vi "Parse Core.vi"(0 "SA Path in":refnum<class "SA 18GHz Path.lvclass">, 5 "Config Row":string[](array[string]), 11 "error in":errorcluster) -> (4 "SA Path out":refnum<class "SA 18GHz Path.lvclass">, 15 "error out":errorcluster)   [LabVIEW 2023, in "RFFixtureCharact.RFPM.lvlib" / "SA 18GHz Path.lvclass"]
uses:
  SA 18GHz Path.lvclass
  C:/srd-semi-rfcal-software/AuxTools/STSRFFixtureCharactUtility/Source/Code Modules/Common/Base Classes/Path/Path.lvclass
  Charact Result Accessor/Scalar/Scalar Charact Result Accessor.lvclass
  C:/srd-semi-rfcal-software/AuxTools/STSRFFixtureCharactUtility/Source/Code Modules/Fixture/RFPM/Charact Result Accessor/Base/Charact Result Accessor.lvclass
  C:/srd-semi-rfcal-software/AuxTools/STSRFFixtureCharactUtility/Source/Code Modules/Common/Result Accessor/Result Accessor.lvclass
  Common/Base Classes/Path/Path.lvclass/Path.ctl
  Common/Base Classes/Path/Properties/Read Date.vi
  Common/Base Classes/Path/Properties/Read Interval.vi
  Common/Data Cache/Settings Dictionary/Setting Keys.vi
  Public/Base Classes/Scalar/SA Abstract Path/SA Abstract Path.lvclass
  Common/RFCalAndFixtureCharact.Common.lvlib
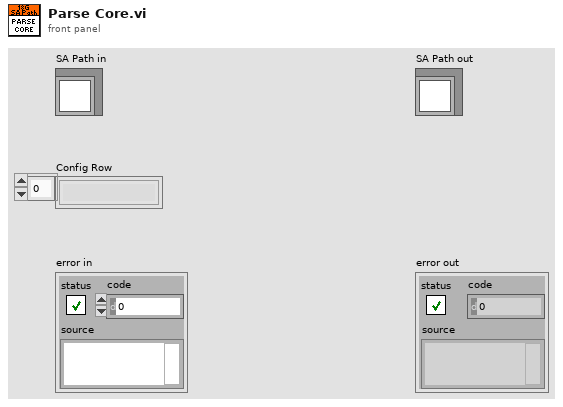
[diagram p1: front panel]
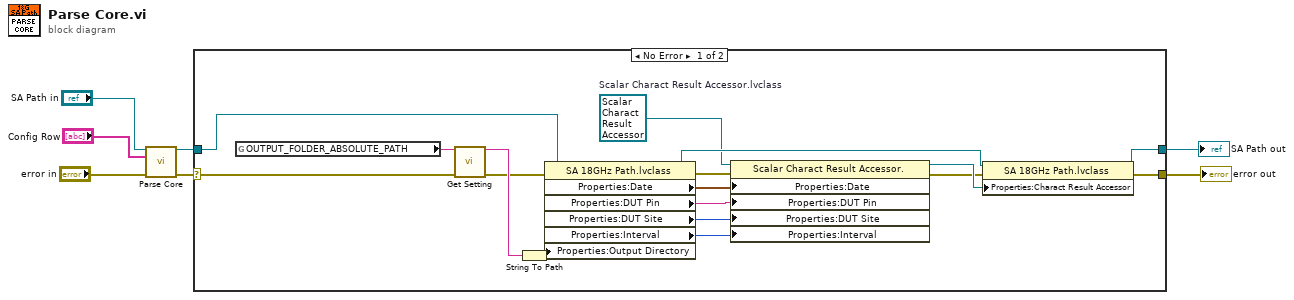
[diagram p0: block diagram]
diagram:
  n1 = call-parent "Parse Core.vi"("SA Path in"="SA Path in", "Config Row"="Config Row", "error in (no error)"="error in") -> ("SA Path out"=w2:refnum<class "SA 18GHz Path.lvclass">, "error out"=w1:errorcluster)  [unwired: 11 in]
  n2 = case shown="No Error" w1 {
    selector: w1 -> [w10 w25]
    tunnel: [w24 w26] -> w6
    tunnel: [w23 w25] -> w4
    tunnel: w2 -> [w13 w26]
    frame No Error {
      w14 = refnum<class "Scalar Charact Result Accessor.lvclass"> refnum  # Scalar Charact Result Accessor.lvclass
      n3 = global read "Setting Keys.vi" "OUTPUT_FOLDER_ABSOLUTE_PATH"() -> (w11:string)
      n4 = call "Get Setting.vi"("Setting name"=w11, "error in (no error)"=w10) -> ("Setting value out"=w12:string, "error out"=w9:errorcluster)  [unwired: 11 in, 1 out]
      n5 = String To Path(string=w12) -> (path=w8:path)
      n6 = property class="SA 18GHz Path.lvclass"(reference=w13, error in=w9, "Properties:Output Directory"=w8) -> (reference out=w21:refnum<class "SA 18GHz Path.lvclass">, error out=w16:errorcluster, "Properties:Date"=w17:timestamp, "Properties:DUT Pin"=w18:string, "Properties:DUT Site"=w19:i32, "Properties:Interval"=w20:i32)
      n7 = property class="Scalar Charact Result Accessor."(reference=w14, error in=w16, "Properties:Date"=w17, "Properties:DUT Pin"=w18, "Properties:DUT Site"=w19, "Properties:Interval"=w20) -> (reference out=w22:refnum<class "Scalar Charact Result Accessor.lvclass">, error out=w15:errorcluster)
      n8 = property class="SA 18GHz Path.lvclass"(reference=w21, error in=w15, "Properties:Charact Result Accessor"=w22) -> (reference out=w24:refnum<class "SA 18GHz Path.lvclass">, error out=w23:errorcluster)
    }
    frame Error {
    }
  }
  "error out" <- w4
  "SA Path out" <- w6
